vi "STM Check Connection.vi"(4 "error in (no error)":errorcluster, 7 "Connection In":refnum<k5>) -> (0 "error out":errorcluster, 2 "Disconnected":bool, 3 "Connection out":refnum<k5>)   [LabVIEW 2010]
doc: "This VI removes the host connection from the manager list if it becomes disconnected for any reason.\n\nCopyright 2015, 2016, 2017 National Instruments Corporation\n\nLicensed under the Apache License, Version 2.0 (the \"License\"); you may not use this file except in compliance with the License.\n\n You may obtain a copy of the License at\n\n http://www.apache.org/licenses/LICENSE-2.0\n\nUnless required by applicable law or agreed to in writing, software distributed under the License is distributed on an \"AS IS\" BASIS, WITHOUT WARRANTIES OR CONDITIONS OF ANY KIND, either express or implied.\n\nSee the License for the specific language governing permissions and limitations under the License."
uses:
  stm_ConnectionMethod.ctl
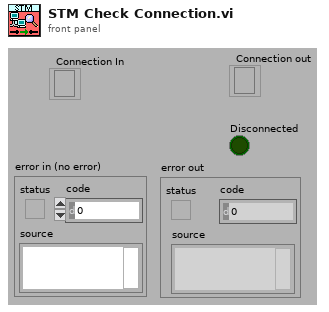
[diagram p1: front panel]
types:
  T1 = typedef "stm_ConnectionMethod.ctl" = enum16{"Initialize", "Add Connection", "Set Properties", "Get Connection(s)", "Close Connection", "Close Connections"}
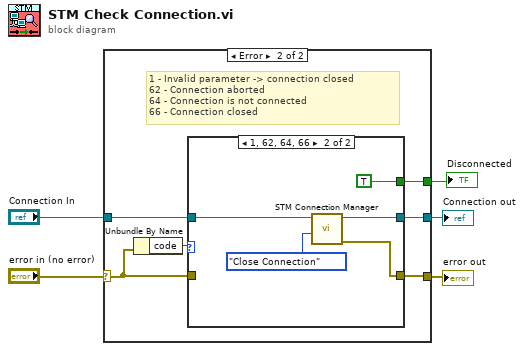
[diagram p0: block diagram]
diagram:
  n1 = case shown="Error" "error in (no error)" {
    selector: "error in (no error)" -> [w7 w12]
    tunnel: [w7 w11] -> w4
    tunnel: "Connection In" -> [w6 w10]
    tunnel: [w6 w9] -> w2
    tunnel: [_ w8] -> w1
    frame No Error {
    }
    frame Error {
      # "1 - Invalid parameter -> connection closed\n62 - Connection aborted\n64 - Connection is not connected\n66 - Connection closed"
      n2 = Unbundle By Name(w12) -> ("code"=w13:i32)
      n3 = case shown="1, 62, 64, 66" w13 {
        tunnel: w12 -> [w15 _]
        tunnel: [w15 w16] -> w11
        tunnel: w10 -> [w14 w20]
        tunnel: [w14 w17] -> w9
        tunnel: [_ TRUE] -> w8
        frame 0, Default {
        }
        frame 1, 62, 64, 66 {
          n4 = call "STM Connection Manager.vi"("Method"=stm_ConnectionMethod."Close Connection", "Connection In"=w20) -> ("error out"=w16:errorcluster, "Connection Out"=w17:refnum<k5>)  [unwired: 3 in, 5 out]
        }
      }
    }
  }
  "error out" <- w4
  "Connection out" <- w2
  "Disconnected" <- w1
